vi "Event Demo Sub Init.vi"(5 "stop":refnum<vi>, 6 "init counter":refnum<vi>, 7 "error in":errorcluster, 8 "max PVs per thread":i32=100, 9 "field names":string[](array[string]), 10 "PV names":string[](array[string])) -> (0 "error out":errorcluster, 1 "number of threads":i32, 2 "references of results":T1(array[cluster]), 3 "subVI References":cluster{refnum<vi>[], refnum<vi>[]})   [LabVIEW 2019]
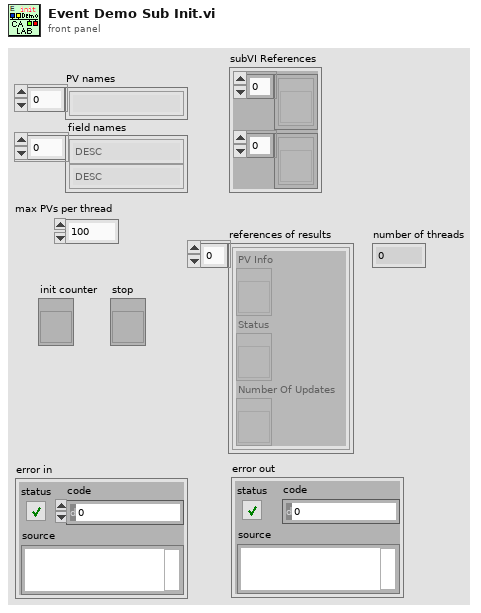
[diagram p1: front panel]
types:
  T1 = cluster{"PV Info":refnum<vi>, "Status":refnum<vi>, "Number Of Updates":refnum<vi>}[]
  T2 = map{string, cluster{"PV Info":refnum<vi>, "Status":refnum<vi>, "Number Of Updates":refnum<vi>}}
  T3 = cluster{"PV Info":refnum<vi>, "Status":refnum<vi>, "Number Of Updates":refnum<vi>}
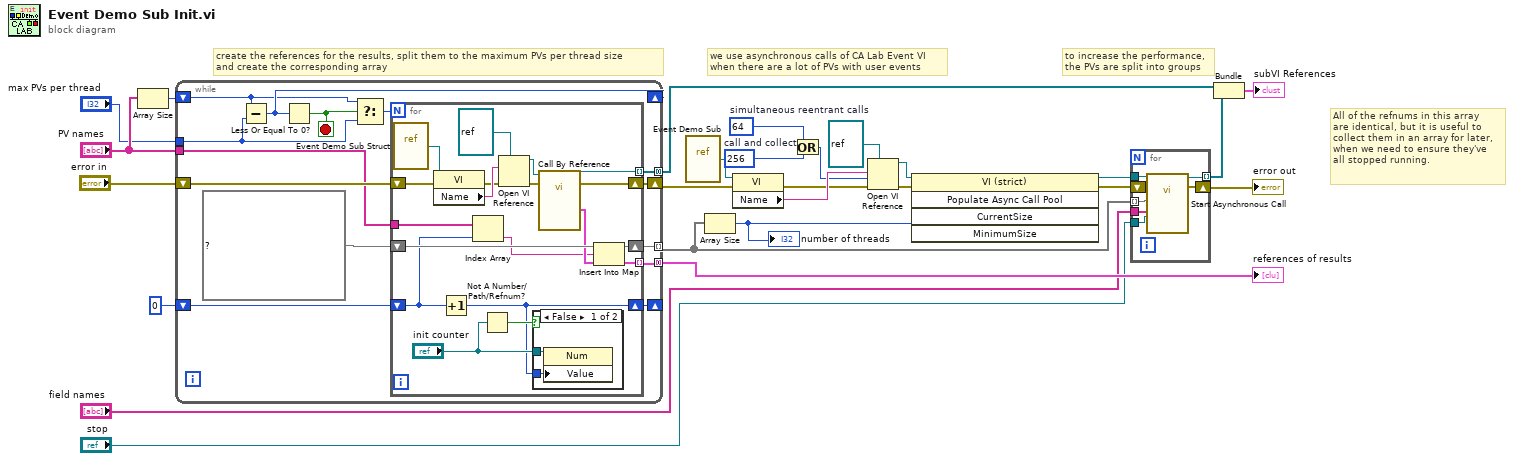
[diagram p0: block diagram]
diagram:
  w16 = 256  # call and collect
  w17 = 64  # simultaneous reentrant calls
  # "All of the refnums in this array\nare identical, but it is useful to\ncollect them in an array for later,\nwhen we need to ensure they've\nall stopped running."
  # "create the references for the results, split them to the maximum PVs per thread size\nand create the corresponding array"
  # "to increase the performance,\nthe PVs are split into groups"
  # "we use asynchronous calls of CA Lab Event VI\nwhen there are a lot of PVs with user events"
  n1 = Array Size(array="PV names") -> (size(s)=w7:i32)
  n2 = while {
    tunnel: [w39] -> w4 mode=concatenating
    shift-right: [w38] -> w2
    shift-left: "error in" -> [w40]
    tunnel: [w37] -> w12 mode=indexing
    shift-right: [w35] -> _
    shift-left: 0 -> [w36]
    shift-right: [w31] -> _
    shift-left: w7 -> [w29]
    tunnel: [w33] -> w11 mode=concatenating
    tunnel: "PV names" -> [w28]
    tunnel: "max PVs per thread" -> [w27]
    stop <- w30 stop-if-true
    n3 = Subtract(x=w29, y=w27) -> (x-y=w31:i32)
    n4 = Less Or Equal To 0?(x=w31) -> (x <= 0?=w30:bool)
    n5 = Select(t=w29, s=w30, f=w27) -> (s? t:f=w32:i32)
    n6 = for {
      N: w32 -> [_]
      tunnel: [w52] -> w39 mode=indexing
      shift-right: [w51] -> w38
      shift-left: w40 -> [w50]
      shift-right: [w49] -> w37
      shift-left: T2 {} ("map in") -> [w48]
      shift-right: [w41] -> w35
      shift-left: w36 -> [w46]
      tunnel: [w47] -> w33 mode=indexing
      tunnel: w28 -> [w44]
      n7 = vi-ref "Event Demo Sub Struct.vi"() -> (w58:refnum<vi>)
      n8 = property class="VI"(reference=w58, error in=w50) -> (error out=w53:errorcluster, "Name"=w57:string)  [unwired: 1 out]
      n9 = Increment(x=w46) -> (x+1=w41:i32)
      n10 = Index Array(array=w44, index=w46) -> (element=w45:string)
      n11 = Not A Number/Path/Refnum?(number/path/refnum="init counter") -> (NaN/Path/Refnum?=w43:bool)
      n12 = Open VI Reference(type specifier VI Refnum (for type only)=refnum<vi> refnum, vi path=w57, error in (no error)=w53) -> (vi reference=w55:refnum<vi>, error out=w54:errorcluster)  [unwired: 3 in]
      n13 = case shown="False" w43 {
        tunnel: "init counter" -> [w60 _]
        tunnel: w41 -> [w59 _]
        frame False {
          n14 = property class="Num"(reference=w60, "Value"=w59) -> ()  [unwired: 1 in, 2 out]
        }
        frame True {
        }
      }
      n15 = call-by-ref "?"(reference=w55, error in=w54) -> (reference out=w52:refnum<vi>, error out=w51:errorcluster, "References"=w47:T3)
      n16 = Insert Into Map(map in=w48, key=w45, value=w47) -> (map out=w49:T2)  [unwired: 2 out]
    }
  }
  "references of results" <- w11
  n17 = vi-ref "Event Demo Sub.vi"() -> (w24:refnum<vi>)
  n18 = Array Size(array=w12) -> (size(s)=w18:i32)
  "number of threads" <- w18
  n19 = property class="VI"(reference=w24, error in=w2) -> (error out=w22:errorcluster, "Name"=w23:string)  [unwired: 1 out]
  n20 = Or(x=w17, y=w16) -> (x .or. y?=w15:i32)
  n21 = Open VI Reference(type specifier VI Refnum (for type only)=refnum<vi> refnum, vi path=w23, options=w15, error in (no error)=w22) -> (vi reference=w19:refnum<vi>, error out=w20:errorcluster)  [unwired: 2 in]
  n22 = invoke class="VI (strict)" method="Populate Async Call Pool"(reference=w19, error in=w20, "MinimumSize"=w18) -> (reference out=w14:refnum<vi>, error out=w13:errorcluster)  [unwired: 2 in, 3 out]
  n23 = for {
    tunnel: w12 -> [w65] mode=indexing
    tunnel: "field names" -> [w64]
    tunnel: "stop" -> [w63]
    shift-right: [w62] -> w10
    shift-left: w13 -> [w66]
    tunnel: w14 -> [w67]
    tunnel: [w61] -> w9 mode=indexing
    n24 = call-by-ref "Start Asynchronous Call"(reference=w67, error in=w66, "Stop reference"=w63, "Field Names"=w64, "map of references"=w65) -> (reference out=w61:refnum<vi>, error out=w62:errorcluster)  [unwired: 9 in]
  }
  "error out" <- w10
  n25 = Bundle(w4, w9) -> (→"subVI References":cluster{refnum<vi>[], refnum<vi>[]})  [unwired: 1 in]
